vi "mm2cntsThorLabs.vi"(11 "XYX cmd [mm]":dbl) -> (3 "XYZ cmd [enc cnts]":dbl)   [LabVIEW 2016]
panel:
  # ">>>"
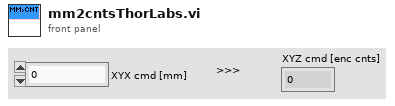
[diagram p1: front panel]
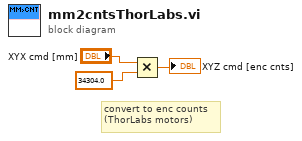
[diagram p0: block diagram]
diagram:
  # "convert to enc counts\n(ThorLabs motors)"
  n1 = Multiply(x="XYX cmd [mm]", y=34304.0) -> (x*y=→"XYZ cmd [enc cnts]":dbl)
